vi "Q_belso.vi"(5 "idolepes":dbl=1.0, 6 "F_belso_fal":dbl, 7 "F_16_17":dbl, 9 "F_belso_vektor":dbl[](array[numeric]), 10 "Q_belso_elozo_vektor":dbl[](array[numeric])) -> (2 "Q_belso_aktualis_vektor":dbl[](array[numeric]))   [LabVIEW 2013]
panel:
  in  "F_belso_vektor":dbl[](array[numeric])
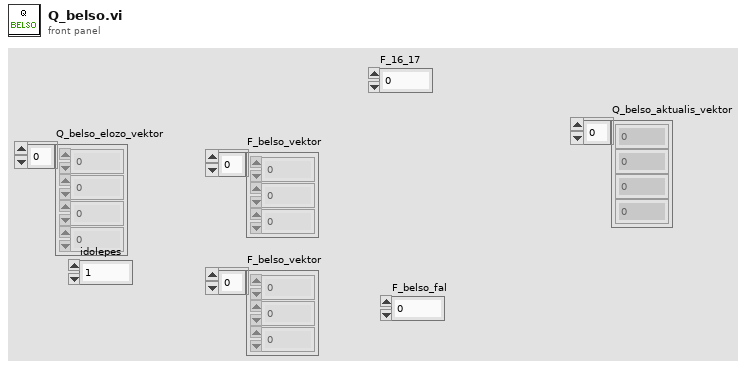
[diagram p1: front panel]
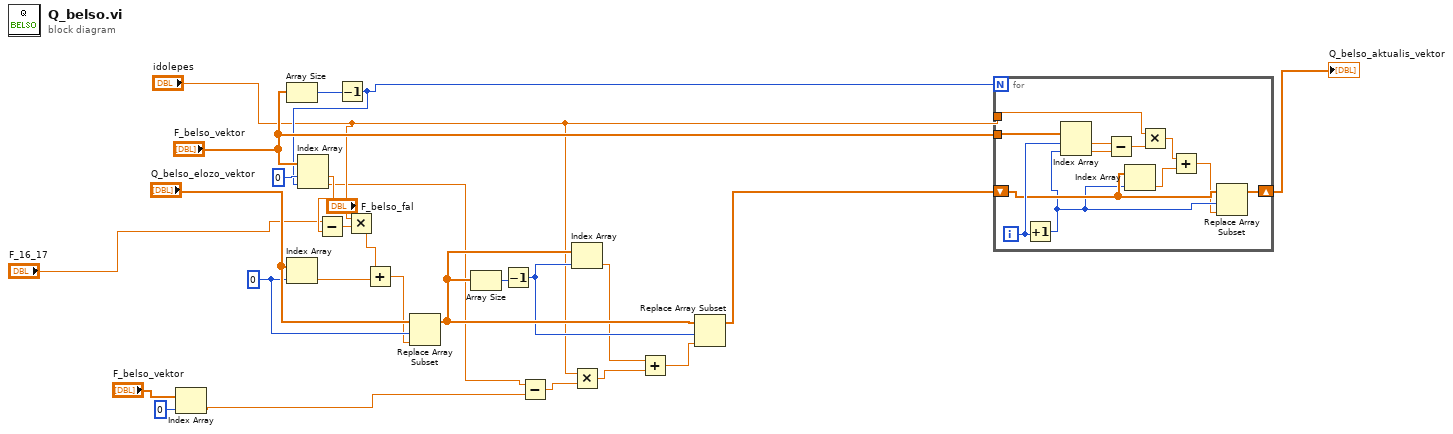
[diagram p0: block diagram]
diagram:
  w16 = 0 ("index")
  n1 = Index Array(array="F_belso_vektor", index=0) -> (element=w2:dbl)
  n2 = Array Size(array="F_belso_vektor") -> (size(s)=w23:i32)
  n3 = Index Array(array="Q_belso_elozo_vektor", index=w16) -> (element=w21:dbl)
  n4 = Decrement(x=w23) -> (x-1=w22:i32)
  n5 = Index Array(array="F_belso_vektor", index #1=0 ("index"), index #2=w22) -> (element #1=w20:dbl, element #2=w5:dbl)
  n6 = Subtract(x="F_16_17", y=w20) -> (x-y=w19:dbl)
  n7 = Multiply(x="idolepes", y=w19) -> (x*y=w18:dbl)
  n8 = Add(x=w18, y=w21) -> (x+y=w15:dbl)
  n9 = Replace Array Subset(array="Q_belso_elozo_vektor", new element=w15, index=w16) -> (w13:dbl[])
  n10 = Array Size(array=w13) -> (size(s)=w12:i32)
  n11 = Decrement(x=w12) -> (x-1=w11:i32)
  n12 = Subtract(x=w5, y=w2) -> (x-y=w6:dbl)
  n13 = Index Array(array=w13, index=w11) -> (element=w9:dbl)
  n14 = Multiply(x="idolepes", y=w6) -> (x*y=w8:dbl)
  n15 = Add(x=w9, y=w8) -> (x+y=w10:dbl)
  n16 = Replace Array Subset(array=w13, new element=w10, index=w11) -> (w14:dbl[])
  n17 = for {
    N: w22 -> [_]
    tunnel: "F_belso_vektor" -> [w38]
    tunnel: "idolepes" -> [w33]
    shift-right: [w27] -> w26
    shift-left: w14 -> [w32]
    i -> [w37]
    n18 = Increment(x=w37) -> (x+1=w31:i32)
    n19 = Index Array(array=w38, index #1=w37, index #2=w31) -> (element #1=w35:dbl, element #2=w36:dbl)
    n20 = Subtract(x=w35, y=w36) -> (x-y=w34:dbl)
    n21 = Index Array(array=w32, index=w31) -> (element=w29:dbl)
    n22 = Multiply(x=w33, y=w34) -> (x*y=w30:dbl)
    n23 = Add(x=w30, y=w29) -> (x+y=w28:dbl)
    n24 = Replace Array Subset(array=w32, new element=w28, index=w31) -> (w27:dbl[])
  }
  "Q_belso_aktualis_vektor" <- w26
